vi "Configure Modulation (Amplitude).vi"(0 "VISA resource name":refnum<visa-resource-name>, 1 "Enable Amplitude Modulation (T: Enable)":bool=TRUE, 5 "Channel (0: Channel 1)":T1 items=["Channel 1", "Channel 2"], 7 "AM Source (0: Internal)":u16(ring) items=["Internal", "External"], 9 "Modulation Waveform (0: Sine)":u16(ring) items=["Sine", "Square", "Triangle", "Ramp", "Down Ramp", "Noise"], 11 "error in (no error)":errorcluster, 12 "Modulation Frequency (1000 Hz)":dbl[unit]=1000.0, 13 "Modulation Depth (0 %)":dbl) -> (4 "VISA resource name out":refnum<visa-resource-name>, 15 "error out":errorcluster)   [LabVIEW 2009, in "Tektronix AFG 3000 Series.lvlib"]
doc: "Configures and enables amplitude modulation (AM). In AM, the amplitude of the carrier is varied by the amplitude of the modulating waveform."
uses:
  Tektronix AFG 3000 Series.lvlib
  controls.llb/Channel.ctl
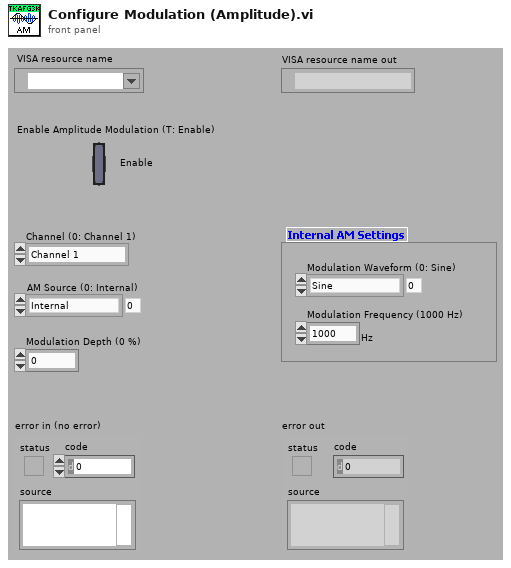
[diagram p1: front panel]
types:
  T1 = typedef "Channel.ctl" = u16
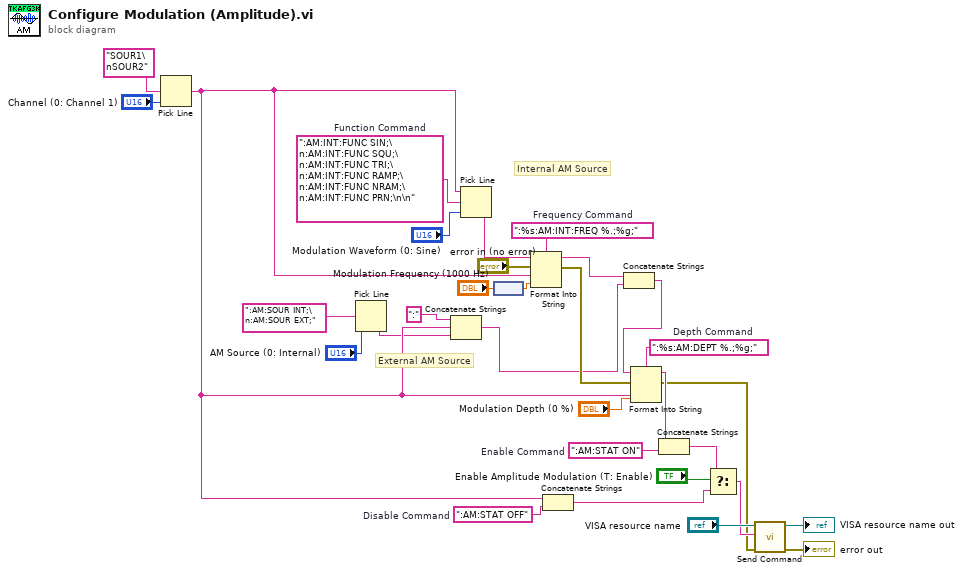
[diagram p0: block diagram]
diagram:
  w20 = ":%s:AM:INT:FREQ %.;%g;"  # Frequency Command
  w21 = ":AM:INT:FUNC SIN;\n:AM:INT:FUNC SQU;\n:AM:INT:FUNC TRI;\n:AM:INT:FUNC RAMP;\n:AM:INT:FUNC NRAM;\n:AM:INT:FUNC PRN;\n\n"  # Function Command
  w25 = ":AM:STAT ON"  # Enable Command
  w27 = ":%s:AM:DEPT %.;%g;"  # Depth Command
  w17 = ":AM:STAT OFF"  # Disable Command
  # "External AM Source"
  # "Internal AM Source"
  n1 = Pick Line(multi-line string="SOUR1\nSOUR2" ("string (\"\")"), line index="Channel (0: Channel 1)") -> (output string=w5:string)  [unwired: 1 out]
  n2 = Pick Line(multi-line string=":AM:SOUR INT;\n:AM:SOUR EXT;" ("Source Command"), line index="AM Source (0: Internal)") -> (output string=w4:string)  [unwired: 1 out]
  n3 = Concatenate Strings(":" ("string"), w5, w4) -> (w1:string)
  n4 = Pick Line(string ("")=w5, multi-line string=w21, line index="Modulation Waveform (0: Sine)") -> (output string=w19:string)
  n5 = node("Modulation Frequency (1000 Hz)") -> (w12:dbl)
  n6 = Format Into String(format string=w20, initial string=w19, error in="error in (no error)", w5, w12) -> (resulting string=w3:string, error out=w14:errorcluster)
  n7 = Concatenate Strings(w5, w17) -> (w16:string)
  n8 = Concatenate Strings(w3, w1) -> (w2:string)
  n9 = Format Into String(format string=w27, initial string=w2, error in=w14, w5, "Modulation Depth (0 %)") -> (resulting string=w26:string, error out=w7:errorcluster)
  n10 = Concatenate Strings(w26, w25) -> (w22:string)
  n11 = Select(t=w22, s="Enable Amplitude Modulation (T: Enable)", f=w16) -> (s? t:f=w8:string)
  n12 = call "Send Command.vi"("error in (no error)"=w7, "write buffer"=w8, "VISA resource name"="VISA resource name") -> ("error out"=→"error out":errorcluster, "VISA resource name out"=→"VISA resource name out":refnum<visa-resource-name>)  [unwired: 7 out]
